vi "Demand to PWM.vi"(11 "Motor Output":dbl) -> (2 "Duty Cycle":dbl, 3 "Direction":bool)   [LabVIEW 2015]
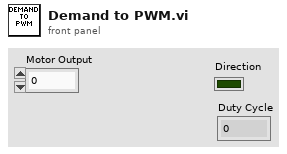
[diagram p1: front panel]
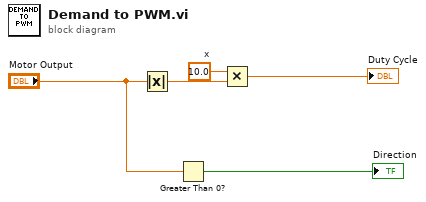
[diagram p0: block diagram]
diagram:
  w4 = 10.0  # x
  n1 = Absolute Value(x="Motor Output") -> (abs(x)=w2:dbl)
  n2 = Greater Than 0?(x="Motor Output") -> (x > 0?=→"Direction":bool)
  n3 = Multiply(x=w4, y=w2) -> (x*y=→"Duty Cycle":dbl)
